vi "DSF.Execution.Builder.New.vi"(8 "error in (no error)":errorcluster, 11 "Plugin Buffer Pools":refnum<class "DSF.Memory.BufferPool.lvclass">[](array[class])) -> (0 "error out":errorcluster, 3 "Builder":refnum<class "DSF.Execution.Builder.lvclass">)   [LabVIEW 2016, in "DSF.Execution.lvlib" / "DSF.Execution.Builder.lvclass"]
uses:
  DSF.Execution.Builder.lvclass
  Memory.BufferPool/DSF.Memory.BufferPool.lvclass
  DSF.Execution.Builder.FIFOs.ctl
  DSF.Execution.Builder.Command FIFO.ctl
  DSF.Execution.Builder.Command Payload.ctl
  DSF.Execution.Builder.Commands.ctl
  DSF.Execution.Builder.Response FIFO.ctl
  DSF.Execution.Builder.Response Payload.ctl
  DSF.Execution.Builder.lvclass/DSF.Execution.Builder.ctl
  DSF.Execution.Builder.Status Pointers.ctl
  Memory.Pointer/DSF.Memory.Pointer.U32.lvclass
  C:/Git/SourceTree/DSF/Source/Submodules/Memory Manager/Source/Classes/Pointer.Internal/Memory.Pointer.Internal.lvclass
  Submodules/Memory Manager/Source/Classes/Pointer.Internal/Methods/Memory.Pointer.Internal.Allocate.vi
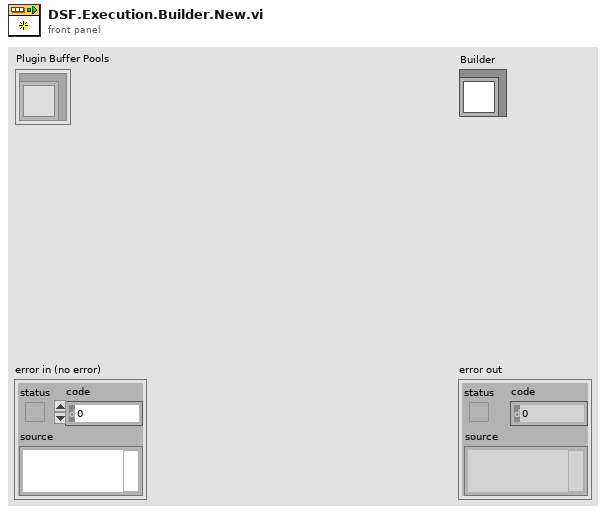
[diagram p1: front panel]
types:
  T1 = typedef "DSF.Execution.lvlib/DSF.Execution.Builder.lvclass/DSF.Execution.Builder.Status Pointers.ctl" = cluster{"Build Duration":refnum<class "DSF.Memory.Pointer.U32.lvclass">}
  T2 = typedef "DSF.Execution.lvlib/DSF.Execution.Builder.lvclass/DSF.Execution.Builder.Response Payload.ctl" = cluster{"command":T3}
  T3 = typedef "DSF.Execution.lvlib/DSF.Execution.Builder.lvclass/DSF.Execution.Builder.Commands.ctl" = enum8{"Initialize", "Build", "Shutdown"}
  T4 = cluster{"read mode":enum16{"polling", "blocking"}, "write mode":enum16{"polling", "blocking"}}
  T5 = typedef "DSF.Execution.lvlib/DSF.Execution.Builder.lvclass/DSF.Execution.Builder.Command Payload.ctl" = cluster{"command":T3, "plugin id":i32, "transfer id":i32}
  T6 = typedef "DSF.Execution.lvlib/DSF.Execution.Builder.lvclass/DSF.Execution.Builder.FIFOs.ctl" = cluster{"Command FIFO":T7, "Response FIFO":T8}
  T7 = typedef "DSF.Execution.lvlib/DSF.Execution.Builder.lvclass/DSF.Execution.Builder.Command FIFO.ctl" = refnum<k33>
  T8 = typedef "DSF.Execution.lvlib/DSF.Execution.Builder.lvclass/DSF.Execution.Builder.Response FIFO.ctl" = refnum<k33>
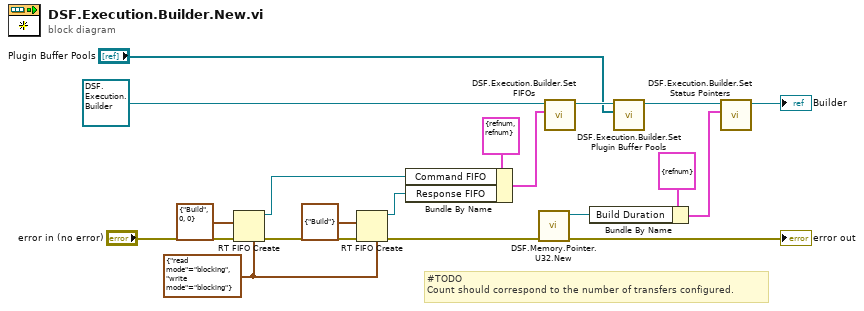
[diagram p0: block diagram]
diagram:
  w10 = T4 {"read mode"=enum."blocking", "write mode"=enum."blocking"} ("r/w modes (polling,polling)")
  # "#TODO\nCount should correspond to the number of transfers configured."
  n1 = RT FIFO Create(1:T5 {"command"=enum."Build", "plugin id"=0, "transfer id"=0} ("Command Payload"), 3:"error in (no error)", 7:w10) -> (8:w8:refnum<k33>, 11:w11:errorcluster)  [unwired: 5 in, 1 out]
  n2 = RT FIFO Create(1:T2 {"command"=enum."Build"} ("Response Payload"), 3:w11, 7:w10) -> (8:w7:refnum<k33>, 11:w5:errorcluster)  [unwired: 5 in, 1 out]
  n3 = Bundle By Name(cluster=T6 {"Command FIFO"=refnum, "Response FIFO"=refnum} ("FIFOs"), "Command FIFO"=w8, "Response FIFO"=w7) -> (w14:T6)
  n4 = call "DSF.Memory.Pointer.U32.New.vi"("error in (no error)"=w5) -> ("error out"=→"error out":errorcluster, "pointer"=w3:refnum<class "DSF.Memory.Pointer.U32.lvclass">)  [unwired: 9 in]
  n5 = call "DSF.Execution.Builder.Set FIFOs.vi"("FIFOs"=w14, "Builder in"=refnum<class "DSF.Execution.Builder.lvclass"> refnum ("Builder")) -> ("Builder out"=w18:refnum<class "DSF.Execution.Builder.lvclass">)  [unwired: 8 in, 1 out]
  n6 = Bundle By Name(cluster=T1 {"Build Duration"=refnum} ("Status Pointers"), "Build Duration"=w3) -> (w2:T1)
  n7 = call "DSF.Execution.Builder.Set Plugin Buffer Pools.vi"("Plugin Buffer Pools"="Plugin Buffer Pools", "Builder in"=w18) -> ("Builder out"=w17:refnum<class "DSF.Execution.Builder.lvclass">)  [unwired: 8 in, 1 out]
  n8 = call "DSF.Execution.Builder.Set Status Pointers.vi"("Status Pointers"=w2, "Builder in"=w17) -> ("Builder out"=→"Builder":refnum<class "DSF.Execution.Builder.lvclass">)  [unwired: 8 in, 1 out]
